vi "Open Window.vi"(10 "Window Name":string) -> (3 "VI输出":refnum<vi>)   [LabVIEW 2018, in "MainInterface.lvlib" / "User Interface.lvclass"]
uses:
  User Interface.lvclass
panel:
  in  "VI引用句柄":refnum<vi>
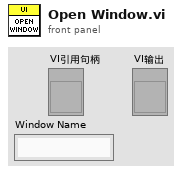
[diagram p1: front panel]
types:
  T1 = enum32{"Invalid", "Standard", "Closed", "Hidden", "Minimized", "Maximized"}
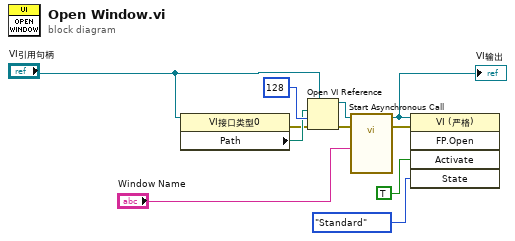
[diagram p0: block diagram]
diagram:
  n1 = property class="VI接口类型0"(reference="VI引用句柄") -> (error out=w8:errorcluster, "Path"=w10:path)  [unwired: 1 in, 1 out]
  n2 = Open VI Reference(type specifier VI Refnum (for type only)="VI引用句柄", vi path=w10, options=128 ("选项"), error in (no error)=w8) -> (vi reference=w9:refnum<vi>, error out=w7:errorcluster)  [unwired: 2 in]
  n3 = call-by-ref "Start Asynchronous Call"(reference=w9, error in=w7, "Window Name"="Window Name") -> (reference out=w6:refnum<vi>, error out=w5:errorcluster)  [unwired: 11 in]
  "VI输出" <- w6
  n4 = invoke class="VI (严格)" method="FP.Open"(reference=w6, error in=w5, "Activate"=TRUE ("激活？"), "State"=T1."Standard" ("状态")) -> ()  [unwired: 1 in, 5 out]
